vi "JSONRPC-GetMethodParams.vi"(8 "error in":errorcluster, 11 "input string":string) -> (0 "error out":errorcluster, 3 "params":string[](array[string]))   [LabVIEW 2013]
doc: "Search for a pair with key 'params' in <b>input string</b> and returns an array containing the params. The VI generates an error if 'params' key does not exist or its value is not an array."
uses:
  <vilib>/regexp/Match Regular Expression.xnode
panel:
  # "GetMethodParams"
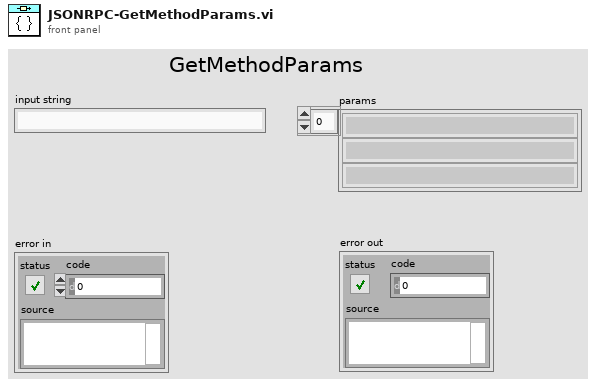
[diagram p1: front panel]
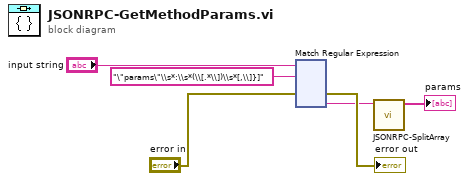
[diagram p0: block diagram]
diagram:
  n1 = xnode "Match Regular Expression"("input string"="input string", "regular expression"="\"params\"\\s*:\\s*(\\[.*\\])\\s*[,\\]}]" ("input string"), "error in"="error in") -> ("error out"=→"error out":errorcluster, "submatch 1"=w3:string)  [unwired: 3 in, 4 out]
  n2 = call "JSONRPC-SplitArray.vi"("input string"=w3) -> ("array"=→"params":string[])  [unwired: 10 in]
